vi "LVClasse_Phase Get Pupil.vi"(0 "Phase in":refnum<class "Phase.lvclass">, 5 "Pupil":refnum<class "Pupil.lvclass">, 11 "error in (no error)":errorcluster) -> (4 "Phase out":refnum<class "Phase.lvclass">, 6 "Pupil (dup)":refnum<class "Pupil.lvclass">, 15 "error out":errorcluster)   [LabVIEW 2020, in "Phase.lvclass"]
doc: "Phase values buffer and pupil getter.\n\n--------------------------------------------------------------------------------\n\n<B>PhaseIn </B> : Phase object.\n<B>PhaseOut </B> : Phase object.\n<B>buffer </B> : Phase values buffer.\n<B>Pupil </B> : pupil object.\n<B>ErrorIn </B> : Error\n<B>ErrorOut </B> : Error\n\n--------------------------------------------------------------------------------"
uses:
  Phase.lvclass
  Pupil.lvclass
  Phase.lvclass/Phase.ctl
  LVClass_Pupil Read Pupil.vi
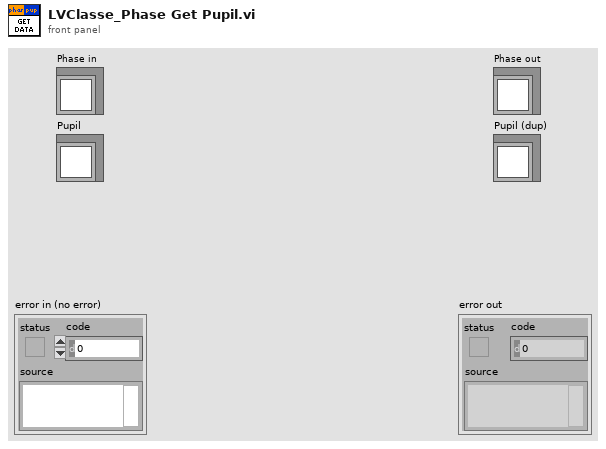
[diagram p1: front panel]
types:
  T1 = typedef "ClassID.ctl" = i64
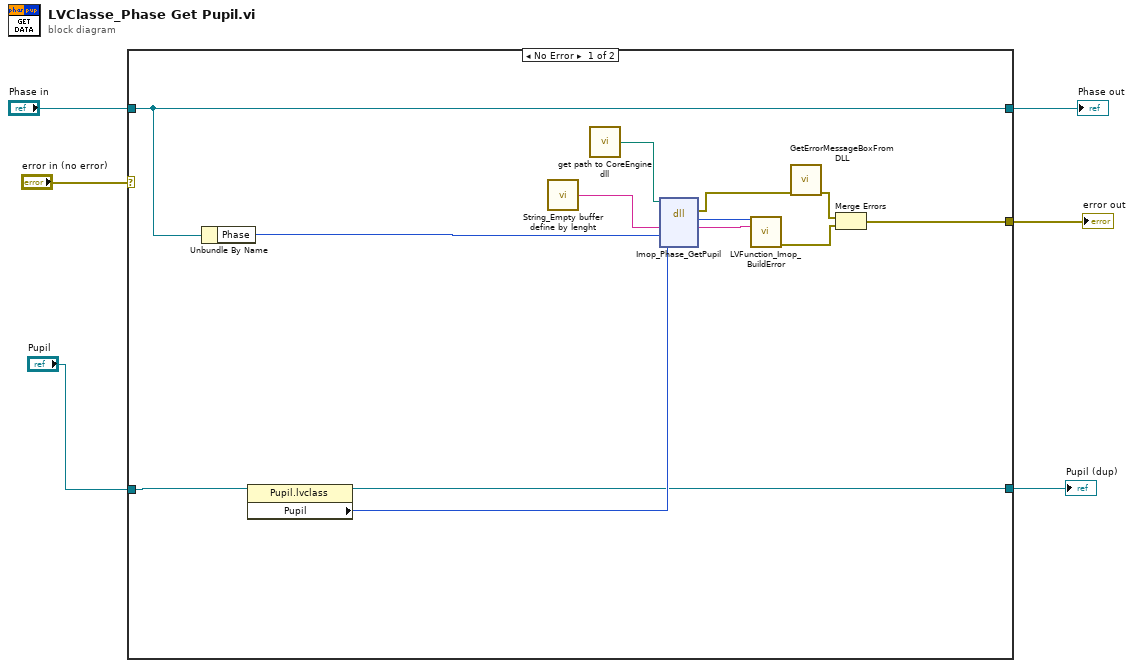
[diagram p0: block diagram]
diagram:
  n1 = case shown="No Error" "error in (no error)" {
    selector: "error in (no error)" -> [_ w22]
    tunnel: [w8 w22] -> w6
    tunnel: [w7 w21] -> w5
    tunnel: "Phase in" -> [w7 w21]
    tunnel: "Pupil" -> [w13 w20]
    tunnel: [w11 w20] -> w3
    frame No Error {
      n2 = Unbundle By Name(w7) -> ("Phase"=w14:T1)
      n3 = property class="Pupil.lvclass"(reference=w13) -> (reference out=w11:refnum<class "Pupil.lvclass">, "Pupil"=w12:T1)  [unwired: 1 in, 1 out]
      n4 = call "String_Empty buffer define by lenght.vi"() -> ("Empty buffer"=w17:string)  [unwired: 1 in]
      n5 = call "get path to CoreEngine dll.vi"() -> ("path to wavekit library"=w16:path)  [unwired: 14 in, 1 out]
      n6 = dll-call lib="D:/2_trunk/Soft_haso/ImOpCoreEngine4_LV2011/DLLs/ImopEngine4_vc100.dll" fn="Imop_Phase_GetPupil"(path in=w16, "message"=w17, "phase"=w14, "pupil"=w12) -> (error out=w15:errorcluster, "return type"=w19:i32, "message"=w18:string)  [unwired: 4 in, 1 out]
      n7 = call "LVFunction_Imop_BuildError.vi"("code"=w19, "String to Prepend to source (\"\")"=w18) -> ("error out"=w9:errorcluster)  [unwired: 13 in]
      n8 = call "GetErrorMessageBoxFromDLL.vi"("error IN"=w15) -> ("error OUT"=w10:errorcluster)  [unwired: 10 in]
      n9 = Merge Errors(w10, w9) -> (w8:errorcluster)
    }
    frame Error {
    }
  }
  "error out" <- w6
  "Phase out" <- w5
  "Pupil (dup)" <- w3
